vi "DigitalIO.vi"(0 "a_hDevice":i32) -> ()   [LabVIEW 2016]
panel:
  in  "Duty7":u8
  in  "Duty6":u8
  in  "Duty5":u8
  in  "Duty3":u8
  in  "Duty2":u8=50
  in  "Duty1":u8
  in  "Freq567":u32
  in  "Freq123":u32
  in  "PWM7":bool
  in  "PWM6":bool
  in  "PWM5":bool
  in  "PWM3":bool
  in  "PWM2":bool
  in  "PWM1":bool
  in  "DO1":bool caption="pin 11"
  in  "DO2":bool caption="pin 2"
  in  "DO3":bool caption="pin 20"
  in  "DO4":bool caption="pin 12"
  in  "DO5":bool caption="pin 3"
  in  "DO6":bool caption="pin 21"
  in  "DO7":bool caption="pin 13"
  in  "DO8":bool caption="pin 4"
  in  "DO9":bool caption="pin 22"
  in  "DO10":bool caption="pin 25"
  out "DI3":bool caption="pin 16"
  out "DI2":bool caption="pin 7"
  out "DI1":bool caption="pin 24"
  in  "GetDigIn":bool
  in  "stop":bool
  # "Digital I/O"
  # "Digital Outputs"
  # "Duty Cycle %"
  # "Frequency (500-300000 Hz)"
  # "Digital Inputs"
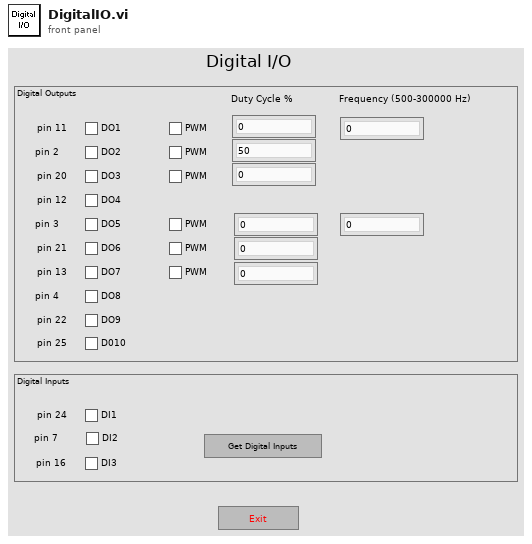
[diagram p1: front panel]
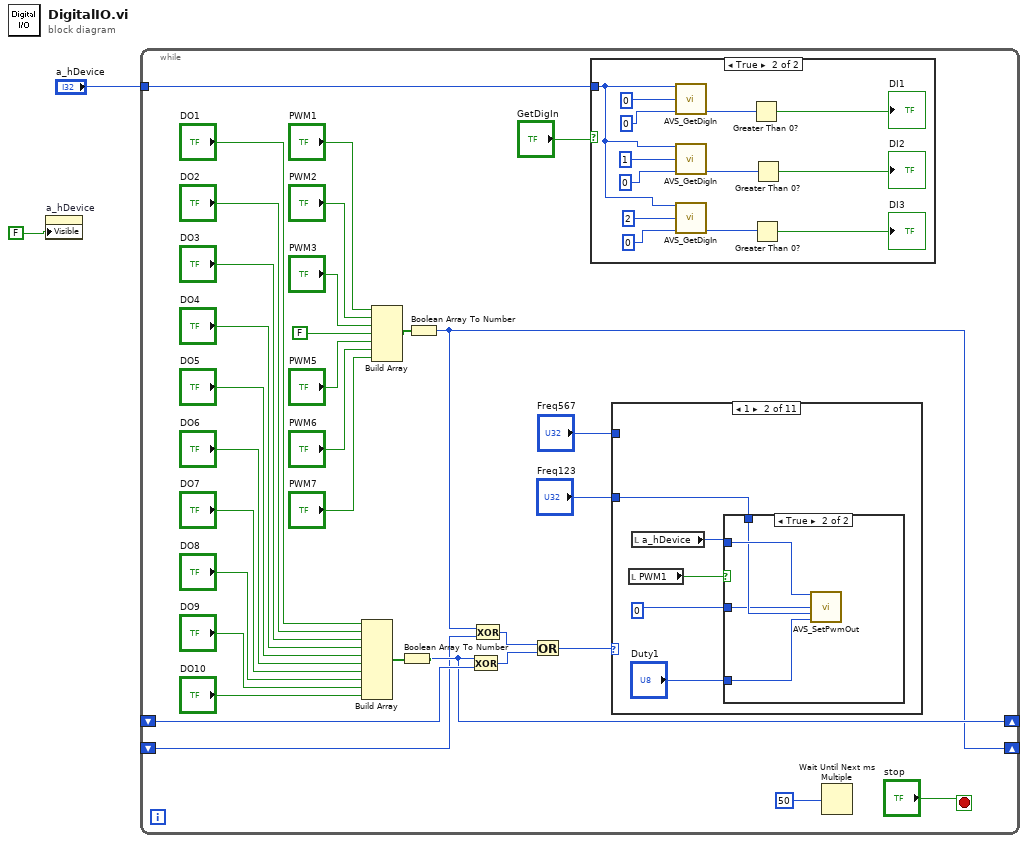
[diagram p0: block diagram]
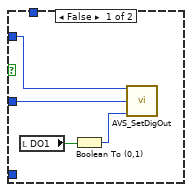
[diagram p3: hidden frame]
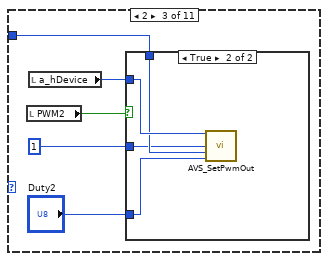
[diagram p4: hidden frame]
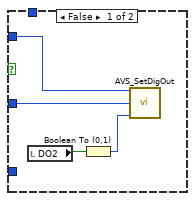
[diagram p5: hidden frame]
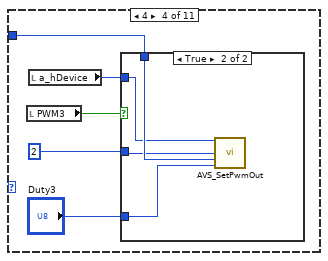
[diagram p6: hidden frame]
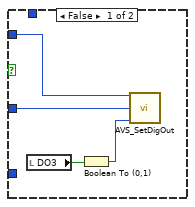
[diagram p7: hidden frame]
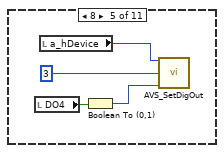
[diagram p8: hidden frame]
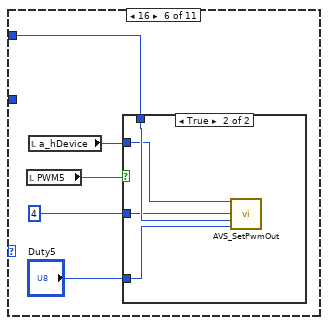
[diagram p9: hidden frame]
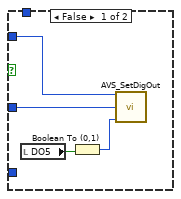
[diagram p10: hidden frame]
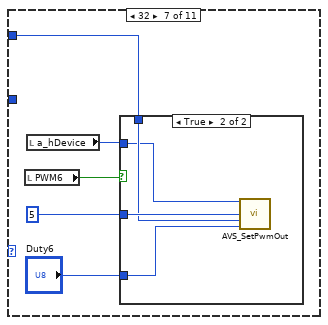
[diagram p11: hidden frame]
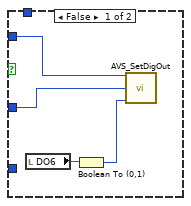
[diagram p12: hidden frame]
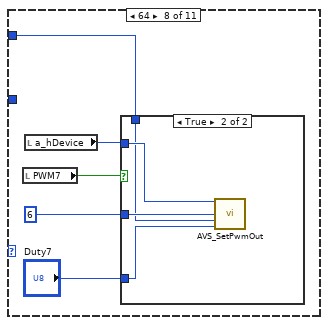
[diagram p13: hidden frame]
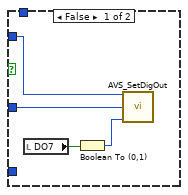
[diagram p14: hidden frame]
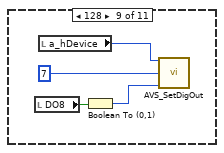
[diagram p15: hidden frame]
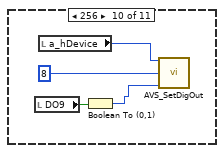
[diagram p16: hidden frame]
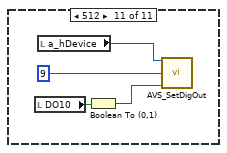
[diagram p17: hidden frame]
diagram:
  n1 = property on="a_hDevice" class="DigNum (strict)"("Visible"=FALSE) -> ()  [unwired: 2 in, 2 out]
  n2 = while {
    tunnel: "a_hDevice" -> [w31]
    shift-right: [w15] -> _
    shift-left: _ -> [w17]
    shift-right: [w9] -> _
    shift-left: _ -> [w7]
    stop <- "stop" stop-if-true
    n3 = Build Array("DO1", "DO2", "DO3", "DO4", "DO5", "DO6", "DO7", "DO8", "DO9", "DO10") -> (w16:bool[])
    n4 = Build Array("PWM1", "PWM2", "PWM3", FALSE, "PWM5", "PWM6", "PWM7") -> (w20:bool[])
    n5 = Boolean Array To Number(Boolean array=w16) -> (number=w15:u32)
    n6 = Boolean Array To Number(Boolean array=w20) -> (number=w9:u32)
    n7 = Exclusive Or(1:w17, 2:w15) -> (0:w10:u32)
    n8 = Exclusive Or(1:w7, 2:w9) -> (0:w11:u32)
    n9 = Or(x=w11, y=w10) -> (x .or. y?=w8:u32)
    n10 = case shown="True" "GetDigIn" {
      tunnel: w31 -> [_ w129]
      frame False {
      }
      frame True {
        n11 = call "AVS_GetDigIn.vi"("a_hDevice"=w129, "a_DigInId"=u8 0 ("a_PortId"), "a_pDigIn"=u8 0 ("a_pAnalogIn")) -> ("a_pDigIn"=w140:u8)  [unwired: 11 in, 1 out]
        n12 = call "AVS_GetDigIn.vi"("a_hDevice"=w129, "a_DigInId"=u8 1 ("a_PortId"), "a_pDigIn"=u8 0 ("a_pAnalogIn")) -> ("a_pDigIn"=w137:u8)  [unwired: 11 in, 1 out]
        n13 = call "AVS_GetDigIn.vi"("a_hDevice"=w129, "a_DigInId"=u8 2 ("a_PortId"), "a_pDigIn"=u8 0 ("a_pAnalogIn")) -> ("a_pDigIn"=w136:u8)  [unwired: 11 in, 1 out]
        n14 = Greater Than 0?(x=w140) -> (x > 0?=→"DI1":bool)
        n15 = Greater Than 0?(x=w136) -> (x > 0?=→"DI3":bool)
        n16 = Greater Than 0?(x=w137) -> (x > 0?=→"DI2":bool)
      }
    }
    n17 = case shown="1" w8 {
      tunnel: "Freq123" -> [_ w38 w51 w64 _ _ _ _ _ _ _]
      tunnel: "Freq567" -> [_ _ _ _ _ w81 w94 w107 _ _ _]
      frame 0, Default {
      }
      frame 1 {
        n18 = local read "PWM1"() -> (w35:bool)
        n19 = local read "a_hDevice"() -> (w37:i32)
        n20 = case shown="True" w35 {
          tunnel: w37 -> [w41 w47]
          tunnel: "Duty1" -> [_ w44]
          tunnel: w38 -> [_ w46]
          tunnel: 0 -> [w40 w45]
          frame False {
            n21 = local read "DO1"() -> (w42:bool)
            n22 = Boolean To (0,1)(Boolean=w42) -> (0, 1=w43:i16)
            n23 = call "AVS_SetDigOut.vi"("a_hDevice"=w41, "a_PortId"=w40, "a_Status"=w43) -> ()  [unwired: 12 in, 1 out]
          }
          frame True {
            n24 = call "AVS_SetPwmOut.vi"("a_hDevice"=w47, "a_PortId"=w45, "a_Freq"=w46, "a_Duty"=w44) -> ()  [unwired: 11 in, 1 out]
          }
        }
      }
      frame 2 {
        n25 = local read "PWM2"() -> (w48:bool)
        n26 = local read "a_hDevice"() -> (w49:i32)
        n27 = case shown="True" w48 {
          tunnel: w49 -> [w56 w59]
          tunnel: "Duty2" -> [_ w60]
          tunnel: w51 -> [_ w58]
          tunnel: 1 -> [w55 w57]
          frame False {
            n28 = local read "DO2"() -> (w54:bool)
            n29 = Boolean To (0,1)(Boolean=w54) -> (0, 1=w53:i16)
            n30 = call "AVS_SetDigOut.vi"("a_hDevice"=w56, "a_PortId"=w55, "a_Status"=w53) -> ()  [unwired: 12 in, 1 out]
          }
          frame True {
            n31 = call "AVS_SetPwmOut.vi"("a_hDevice"=w59, "a_PortId"=w57, "a_Freq"=w58, "a_Duty"=w60) -> ()  [unwired: 11 in, 1 out]
          }
        }
      }
      frame 4 {
        n32 = local read "PWM3"() -> (w61:bool)
        n33 = local read "a_hDevice"() -> (w63:i32)
        n34 = case shown="True" w61 {
          tunnel: "Duty3" -> [_ w73]
          tunnel: w64 -> [_ w72]
          tunnel: w63 -> [w67 w70]
          tunnel: 2 -> [w66 w71]
          frame False {
            n35 = local read "DO3"() -> (w68:bool)
            n36 = Boolean To (0,1)(Boolean=w68) -> (0, 1=w69:i16)
            n37 = call "AVS_SetDigOut.vi"("a_hDevice"=w67, "a_PortId"=w66, "a_Status"=w69) -> ()  [unwired: 12 in, 1 out]
          }
          frame True {
            n38 = call "AVS_SetPwmOut.vi"("a_hDevice"=w70, "a_PortId"=w71, "a_Freq"=w72, "a_Duty"=w73) -> ()  [unwired: 11 in, 1 out]
          }
        }
      }
      frame 8 {
        n39 = local read "DO4"() -> (w75:bool)
        n40 = local read "a_hDevice"() -> (w77:i32)
        n41 = Boolean To (0,1)(Boolean=w75) -> (0, 1=w74:i16)
        n42 = call "AVS_SetDigOut.vi"("a_hDevice"=w77, "a_PortId"=3, "a_Status"=w74) -> ()  [unwired: 12 in, 1 out]
      }
      frame 16 {
        n43 = local read "PWM5"() -> (w78:bool)
        n44 = local read "a_hDevice"() -> (w80:i32)
        n45 = case shown="True" w78 {
          tunnel: w80 -> [w86 w88]
          tunnel: 4 -> [w85 w87]
          tunnel: "Duty5" -> [_ w90]
          tunnel: w81 -> [_ w89]
          frame False {
            n46 = local read "DO5"() -> (w84:bool)
            n47 = Boolean To (0,1)(Boolean=w84) -> (0, 1=w83:i16)
            n48 = call "AVS_SetDigOut.vi"("a_hDevice"=w86, "a_PortId"=w85, "a_Status"=w83) -> ()  [unwired: 12 in, 1 out]
          }
          frame True {
            n49 = call "AVS_SetPwmOut.vi"("a_hDevice"=w88, "a_PortId"=w87, "a_Freq"=w89, "a_Duty"=w90) -> ()  [unwired: 11 in, 1 out]
          }
        }
      }
      frame 32 {
        n50 = local read "PWM6"() -> (w91:bool)
        n51 = local read "a_hDevice"() -> (w92:i32)
        n52 = case shown="True" w91 {
          tunnel: w92 -> [w99 w100]
          tunnel: 5 -> [w98 w102]
          tunnel: "Duty6" -> [_ w103]
          tunnel: w94 -> [_ w101]
          frame False {
            n53 = local read "DO6"() -> (w96:bool)
            n54 = Boolean To (0,1)(Boolean=w96) -> (0, 1=w97:i16)
            n55 = call "AVS_SetDigOut.vi"("a_hDevice"=w99, "a_PortId"=w98, "a_Status"=w97) -> ()  [unwired: 12 in, 1 out]
          }
          frame True {
            n56 = call "AVS_SetPwmOut.vi"("a_hDevice"=w100, "a_PortId"=w102, "a_Freq"=w101, "a_Duty"=w103) -> ()  [unwired: 11 in, 1 out]
          }
        }
      }
      frame 64 {
        n57 = local read "PWM7"() -> (w104:bool)
        n58 = local read "a_hDevice"() -> (w105:i32)
        n59 = case shown="True" w104 {
          tunnel: w105 -> [w112 w114]
          tunnel: 6 -> [w111 w116]
          tunnel: "Duty7" -> [_ w115]
          tunnel: w107 -> [_ w113]
          frame False {
            n60 = local read "DO7"() -> (w110:bool)
            n61 = Boolean To (0,1)(Boolean=w110) -> (0, 1=w109:i16)
            n62 = call "AVS_SetDigOut.vi"("a_hDevice"=w112, "a_PortId"=w111, "a_Status"=w109) -> ()  [unwired: 12 in, 1 out]
          }
          frame True {
            n63 = call "AVS_SetPwmOut.vi"("a_hDevice"=w114, "a_PortId"=w116, "a_Freq"=w113, "a_Duty"=w115) -> ()  [unwired: 11 in, 1 out]
          }
        }
      }
      frame 128 {
        n64 = local read "DO8"() -> (w118:bool)
        n65 = local read "a_hDevice"() -> (w120:i32)
        n66 = Boolean To (0,1)(Boolean=w118) -> (0, 1=w117:i16)
        n67 = call "AVS_SetDigOut.vi"("a_hDevice"=w120, "a_PortId"=7, "a_Status"=w117) -> ()  [unwired: 12 in, 1 out]
      }
      frame 256 {
        n68 = local read "DO9"() -> (w122:bool)
        n69 = local read "a_hDevice"() -> (w124:i32)
        n70 = Boolean To (0,1)(Boolean=w122) -> (0, 1=w121:i16)
        n71 = call "AVS_SetDigOut.vi"("a_hDevice"=w124, "a_PortId"=8, "a_Status"=w121) -> ()  [unwired: 12 in, 1 out]
      }
      frame 512 {
        n72 = local read "DO10"() -> (w126:bool)
        n73 = local read "a_hDevice"() -> (w128:i32)
        n74 = Boolean To (0,1)(Boolean=w126) -> (0, 1=w125:i16)
        n75 = call "AVS_SetDigOut.vi"("a_hDevice"=w128, "a_PortId"=9, "a_Status"=w125) -> ()  [unwired: 12 in, 1 out]
      }
    }
    n76 = Wait Until Next ms Multiple(millisecond multiple=u32 50) -> ()  [unwired: 1 out]
  }
